vi "Generate Application Call Error.vi"() -> (0 "error out":errorcluster)   [LabVIEW 2019, in "SEECD System Explorer.lvlib"]
uses:
  SEECD System Explorer.lvlib
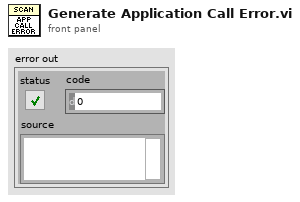
[diagram p1: front panel]
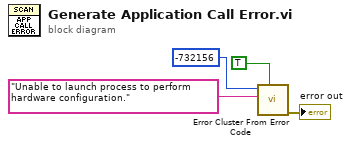
[diagram p0: block diagram]
diagram:
  n1 = call <vilib>:"Error Cluster From Error Code.vi"("show call chain? (False)"=TRUE, "error message (\"\")"="Unable to launch process to perform hardware configuration." ("source"), "error code (0)"=-732156 ("code")) -> ("error out"=→"error out":errorcluster)  [unwired: 6 in]
